vi "4Pi Dual DM - Mode Scan Engine.vi"() -> ()   [LabVIEW 2016]
uses:
  <vilib>/vision/Image Controls.llb/IMAQ Image.ctl
  Hardware Configuration/Hardware Configuration Controls/Device Type.ctl
  Hardware Configuration/Hardware Configuration Controls/Device Function.ctl
  4Pi Dual DM - Controls/4Pi Dual DM - Standard Action.ctl
  4Pi Dual DM - Controls/4Pi Dual DM - Standard Counter Action.ctl
  <vilib>/Analysis/baseanly.llb/Mean (DBL).vi
  <vilib>/Analysis/NI_AALBase.lvlib
  <vilib>/Analysis/NI_AALPro.lvlib
  <vilib>/Analysis/6fits.llb/Curve Fitting Criteria.ctl
  <vilib>/gmath/NI_Gmath.lvlib
panel:
  in  "Image Delay":u32=1
  in  "Accums":u16=1
  in  "Initial Guess":T1={"Amp"=7.0, "Center"=7.0, "Sigma"=7.0, "Offset"=7.0}
  in  "Manual Initial Guess":bool
  in  "Upper Limit":dbl=7.0
  in  "Lower Limit":dbl=7.0
  out "Metric":cluster{dbl[], dbl[]}[](graph)
  out "Image":u16[][](graph)
  in  "Step Size (nm)":u16=7
  in  "Number of Steps":u16=7
  in  "Get Image":bool
  in  "Scan Next Mode":bool
  in  "Metric":u16(ring) items=["Max Intensity", "No Zero Mean", "Threshold Mean"]
  in  "Fit Type":u16(ring) items=["Guassian", "Quadratic"]
  in  "Mode":i32(ring) items=["1", "2", "3", "4", "5", "6", "7", "8", "9", "10", "11", "12", "13", "14", "15", "16", "17", "18", "19", "20", "21", "22", "23", "24", "25", "26", "27", "28", "29", "30", "31", "32", "33", "34", "35", "36", "37", "38", "39", "40", "41", "42", "43", "44", "45", "46", "47", "48", "49", "50", "51", "52", "53", "54", "55", "56", "57", "58", "59", "60", "61", "62", "63", "64", "65", "66", "67", "68", "69", "70", "71", "72", "73", "74", "75", "76", "77", "78", "79", "80", "81", "82", "83", "84", "85", "86", "87", "88", "89", "90", "91", "92", "93", "94", "95", "96", "97", "98", "99", "100", "101", "102", "103", "104", "105", "106", "107", "108", "109", "110", "111", "112", "113", "114", "115", "116", "117", "118", "119", "120", "121", "122", "123", "124", "125", "126", "127", "128", "129", "130", "131", "132", "133", "134", "135", "136", "137", "138", "139", "140", "<141>", "<142>", "<143>", "<144>"]
  in  "Apply":bool
  in  "Fit Data":bool
  in  "Scan Mode":bool
  in  "Exit":bool
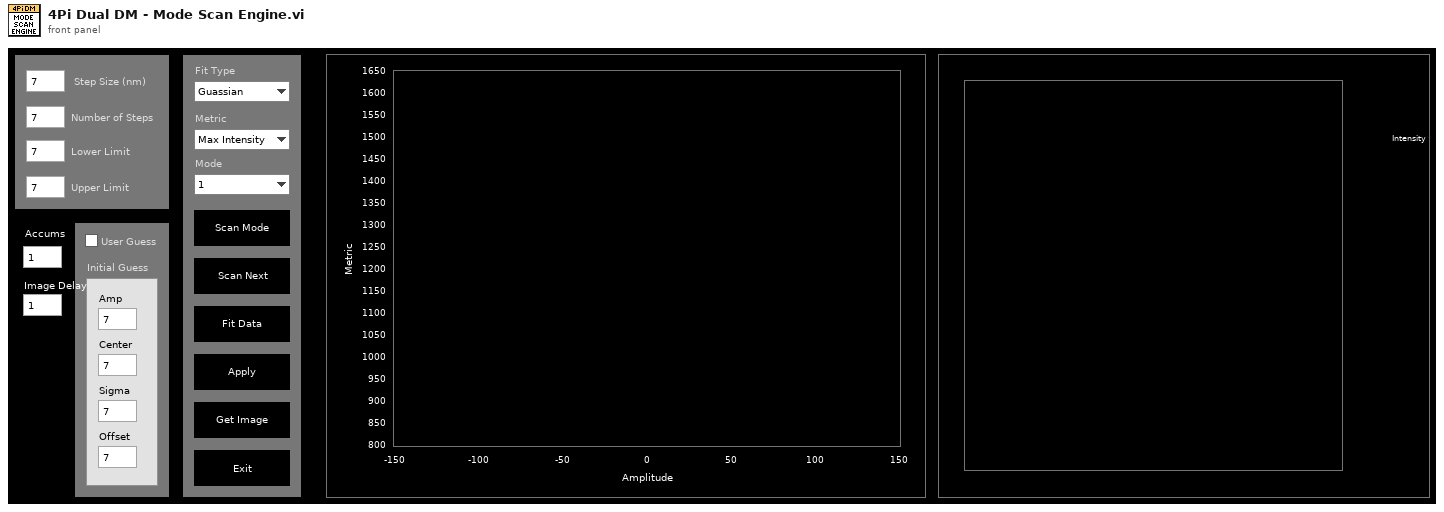
[diagram p1: front panel]
types:
  T1 = cluster{"Amp":dbl, "Center":dbl, "Sigma":dbl, "Offset":dbl}
  T2 = typedef "Device Function.ctl" = enum16{"Primary", "Secondary", "Overview", "Wide Field Drift Correction", "642 nm Excitation", "560 nm Excitation", "546 nm Excitation", "488 nm Excitation", "405 nm Excitation", "Objective Drift Correction", "Objective XY", "Objective Z", "Sample XY", "Sample Coarse Z", "Sample Z", "4Pi Lower", "4Pi Upper", "Adj Cavity"}
  T3 = typedef "Device Type.ctl" = enum16{"AOTF", "Camera", "Deformable Mirror", "Laser", "Shutter", "Stage"}
  T4 = typedef "IMAQ Image.ctl" = refnum<image>
  T5 = typedef "4Pi Dual DM - Standard Action.ctl" = enum16{"Read", "Write"}
  T6 = typedef "4Pi Dual DM - Standard Counter Action.ctl" = enum16{"Initialize", "Update Count", "Get Count"}
  T7 = cluster{"amp min":dbl, "amp max":dbl, "center min":dbl, "center max":dbl, "deviation min":dbl, "deviation max":dbl, "offset min":dbl, "offset max":dbl}
  T8 = enum16{"Linear", "Polynomial", "Exponential", "Power"}
  T9 = typedef "4Pi Dual DM - Mirror Modes DUAL.ctl" = cluster{"Mode":string, "Amplitude":dbl}[][]
  T10 = cluster{"Amplitude Out":dbl[], "Metric Out":dbl[]}
  T11 = cluster{"Amp":dbl, "Numeric":dbl, "Sigma":dbl, "Offset":dbl}
  T12 = typedef "NI_AALPro.lvlib/Curve Fitting Criteria.ctl" = u16
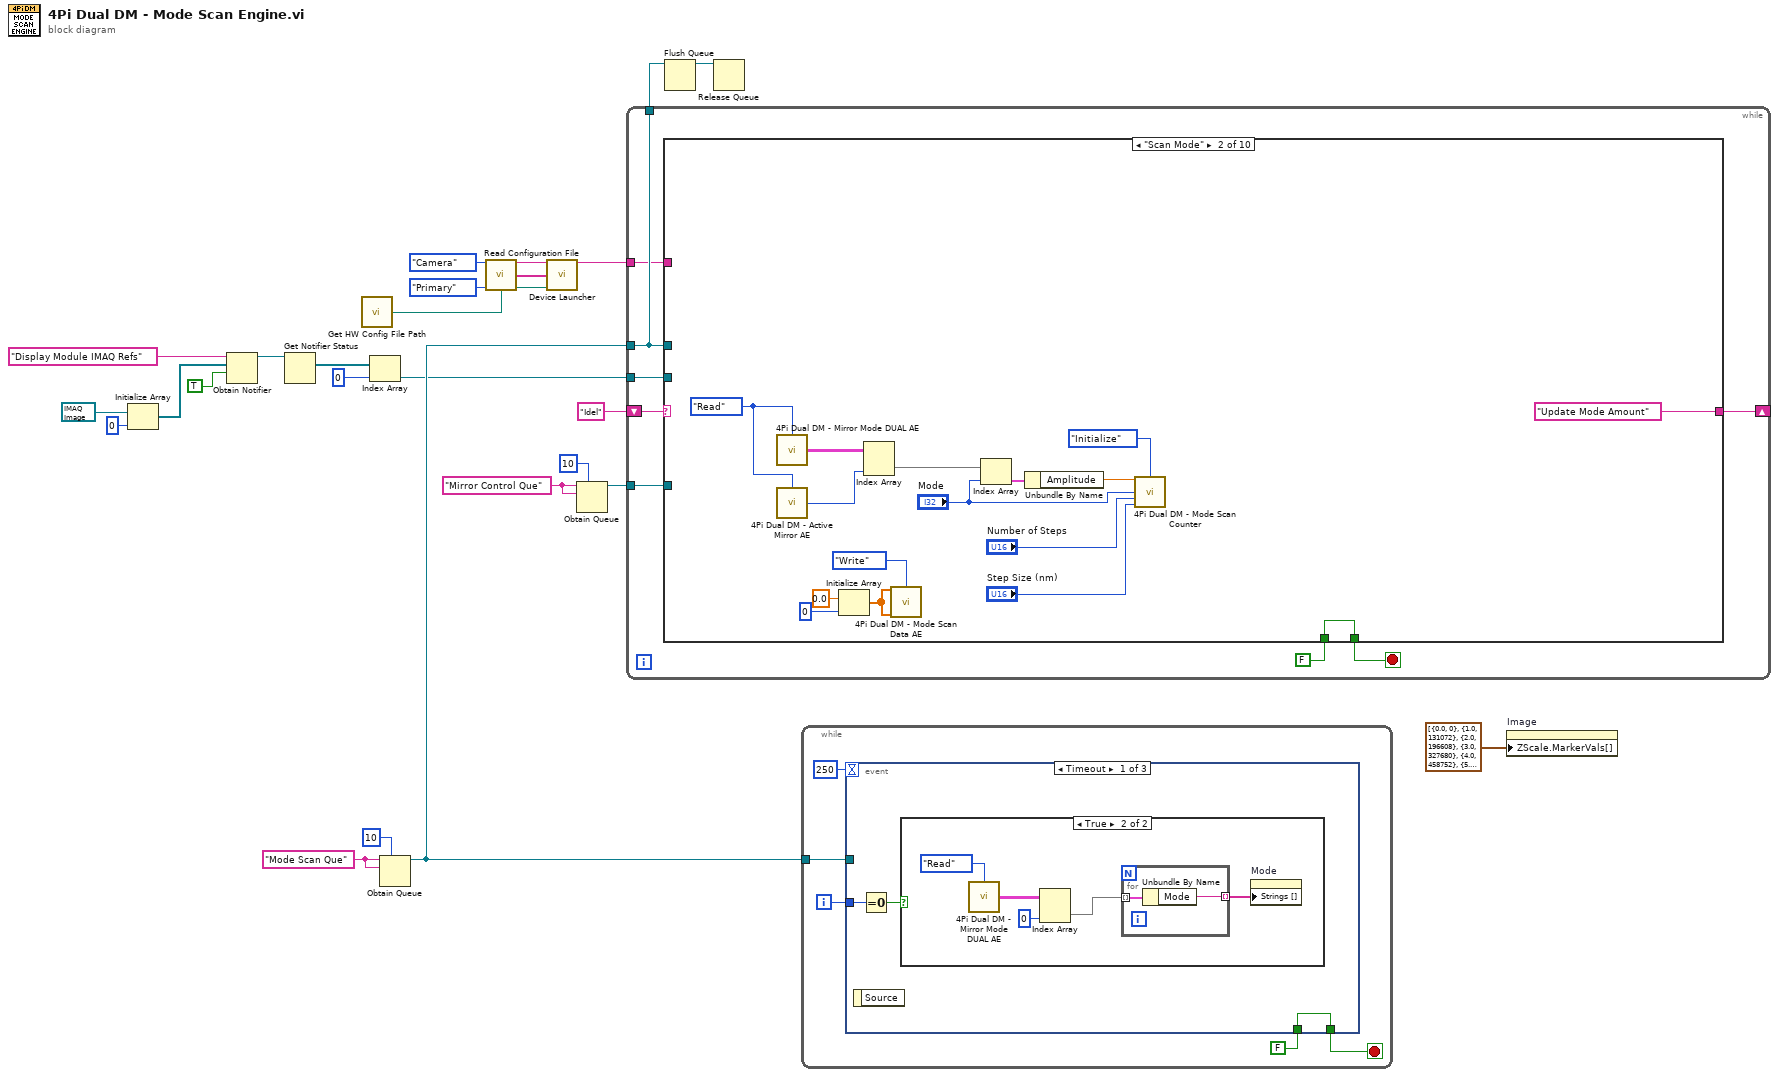
[diagram p0: block diagram]
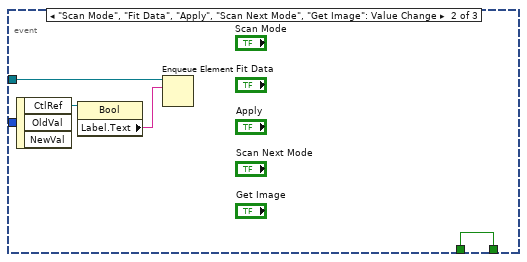
[diagram p3: hidden frame]
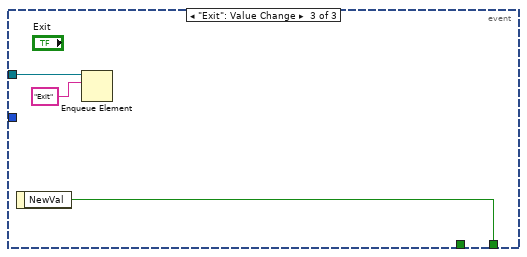
[diagram p4: hidden frame]
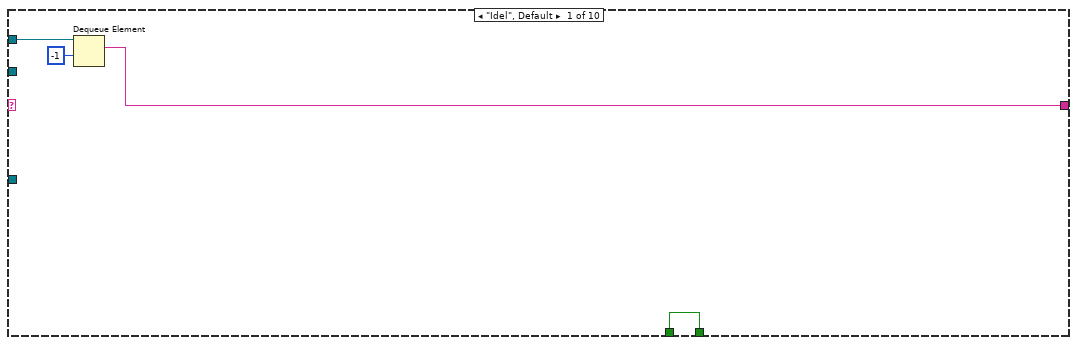
[diagram p5: hidden frame]
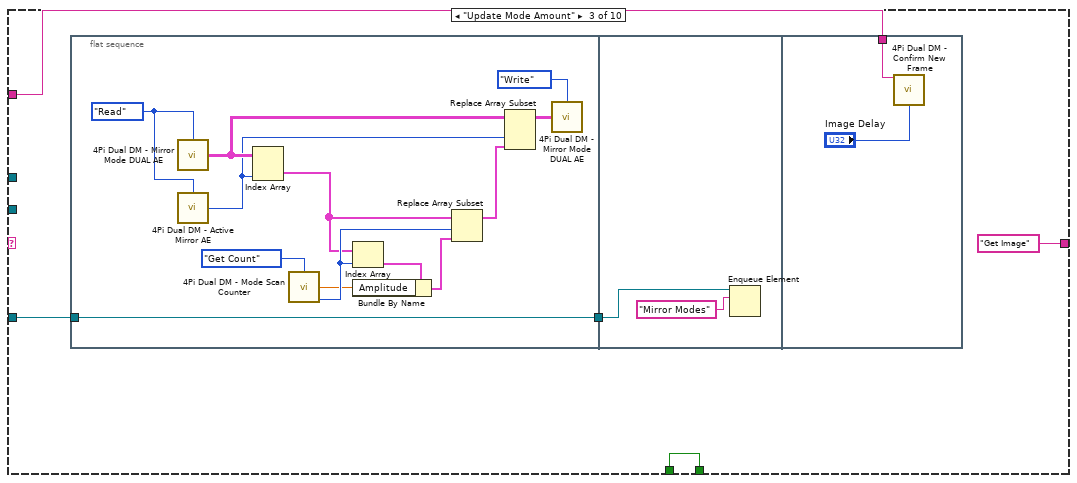
[diagram p6: hidden frame]
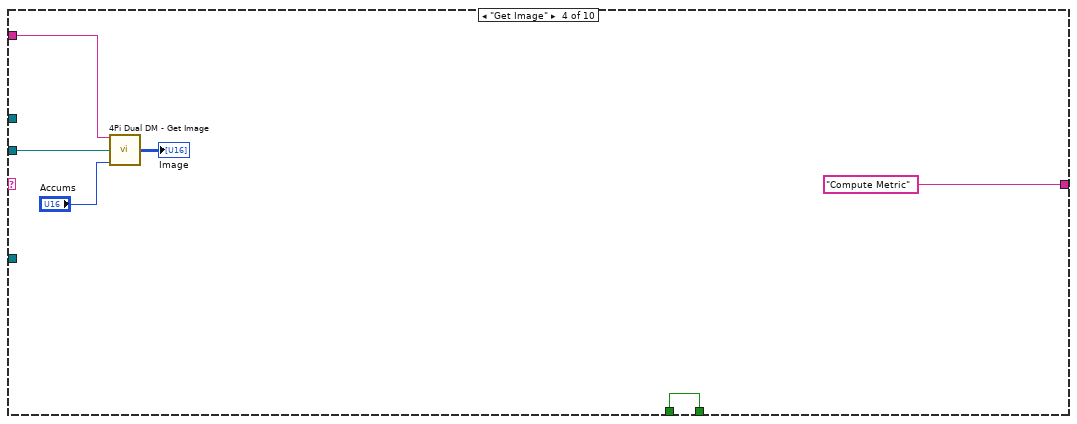
[diagram p7: hidden frame]
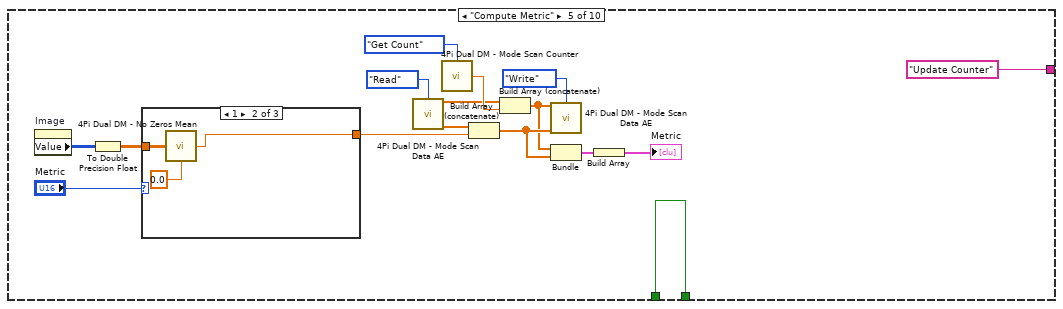
[diagram p8: hidden frame]
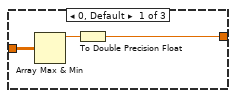
[diagram p9: hidden frame]
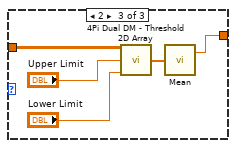
[diagram p10: hidden frame]
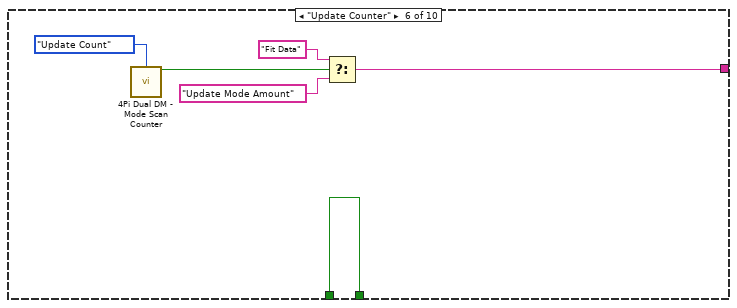
[diagram p11: hidden frame]
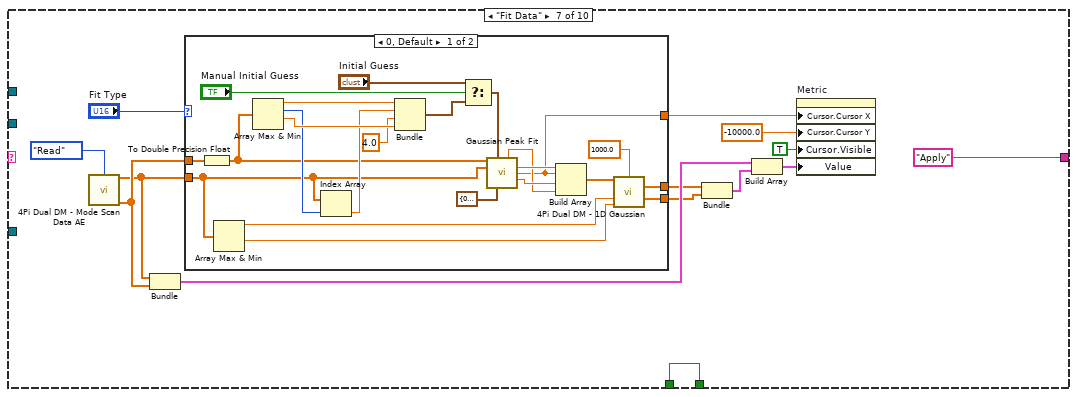
[diagram p12: hidden frame]
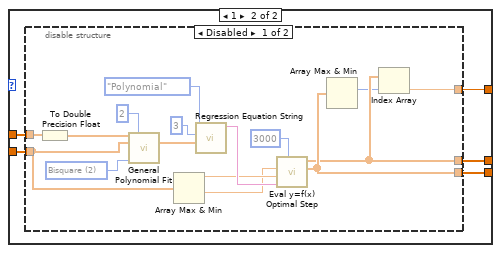
[diagram p13: hidden frame]
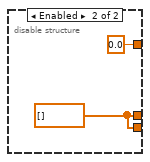
[diagram p14: hidden frame]
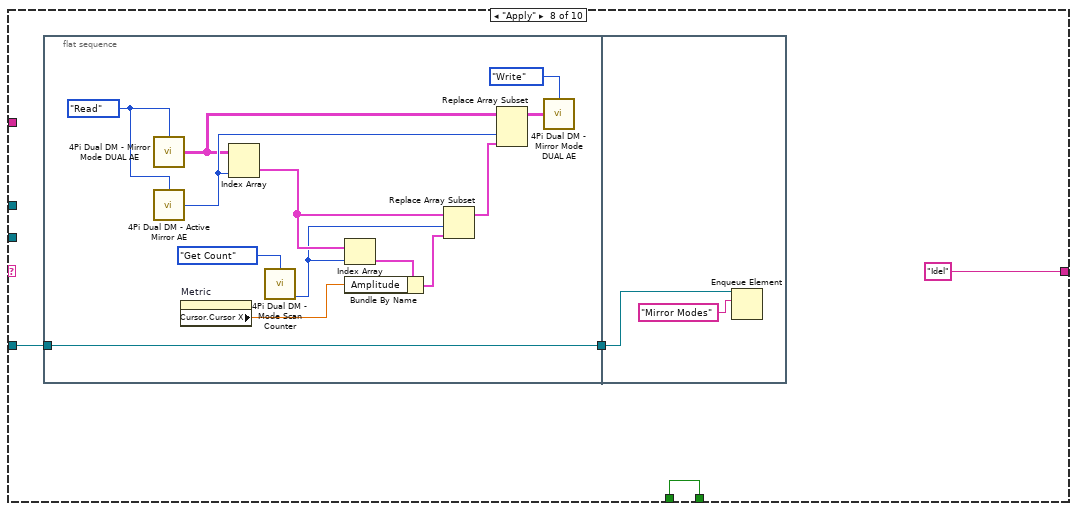
[diagram p15: hidden frame]
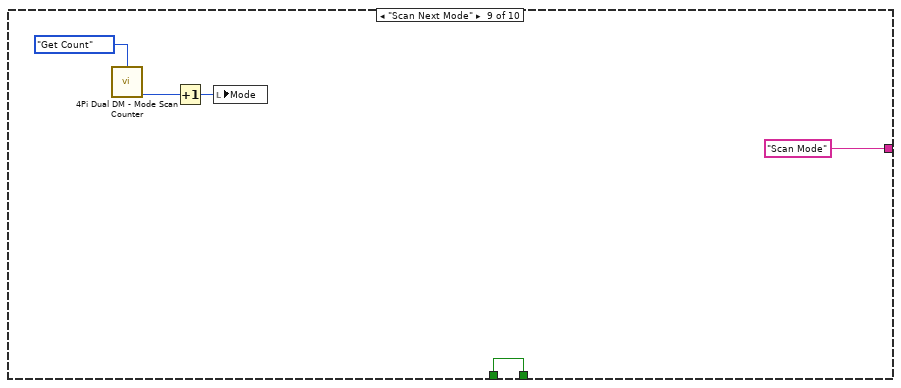
[diagram p16: hidden frame]
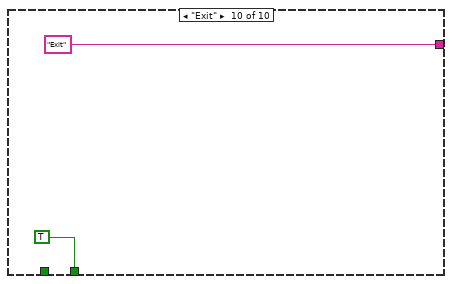
[diagram p17: hidden frame]
diagram:
  w20 = "Mirror Control Que" ("name (unnamed)")
  w25 = "Mode Scan Que" ("name (unnamed)")
  n1 = Initialize Array(T4 refnum ("New Image"), 0 ("dimension size")) -> (w12:T4[])
  n2 = Obtain Notifier(name (unnamed)="Display Module IMAQ Refs", notification data type=w12, create if not found? (T)=TRUE) -> (notifier out=w11:refnum<notifier>)  [unwired: 1 in, 2 out]
  n3 = Get Notifier Status(notifier=w11) -> (current notification=w10:T4[])  [unwired: 1 in, 4 out]
  n4 = call "Get HW Config File Path.vi"() -> ("File Path"=w2:path)  [unwired: 14 in, 1 out]
  n5 = Index Array(array=w10, index=0) -> (element=w8:T4)
  n6 = Obtain Queue(max queue size (-1, unlimited)=10, name (unnamed)=w25, element data type=w25) -> (queue out=w23:refnum<queue>)  [unwired: 2 in, 2 out]
  n7 = call "Read Configuration File.vi"("Device Type"=Device_Type."Camera", "Device Function"=Device_Function."Primary", "Config File Path"=w2) -> ("Unique Notifier Name"=w3:string, "Device Ports/IDs/Channels"=w5:string[], "Device Engine Path"=w4:path)  [unwired: 9 in, 1 out]
  n8 = call "Device Launcher.vi"("Notifier Name"=w3, "Device Ports/IDs/Channels"=w5, "Device Engine Path"=w4) -> ("Notifier Name"=w1:string)  [unwired: 11 in, 1 out]
  n9 = Obtain Queue(max queue size (-1, unlimited)=10, name (unnamed)=w20, element data type=w20) -> (queue out=w18:refnum<queue>)  [unwired: 2 in, 2 out]
  n10 = while {
    shift-right: [w31] -> _
    shift-left: "Idel" -> [w34]
    tunnel: w23 -> [w30]
    tunnel: [w30] -> w22
    tunnel: w18 -> [w29]
    tunnel: w8 -> [w28]
    tunnel: w1 -> [w27]
    stop <- w33 stop-if-true
    n11 = case shown="\"Scan Mode\"" w34 {
      tunnel: [w38 w54 w59 w82 w97 w115 w129 w179 w199 TRUE] -> w33
      tunnel: FALSE -> [w38 w54 w59 w82 w97 w115 w129 w179 w199 _]
      tunnel: w30 -> [w36 _ _ _ _ _ _ _ _ _]
      tunnel: [w35 "Update Mode Amount" ("name (unnamed)") "Get Image" ("name (unnamed)") "Compute Metric" ("name (unnamed)") "Update Counter" ("name (unnamed)") w112 "Apply" ("name (unnamed)") "Idel" ("name (unnamed)") "Scan Mode" ("name (unnamed)") "Exit" ("name (unnamed)")] -> w31
      tunnel: w29 -> [_ _ w58 _ _ _ _ w177 _ _]
      tunnel: w28 -> [_ _ _ w79 _ _ _ _ _ _]
      tunnel: w27 -> [_ _ w55 w78 _ _ _ _ _ _]
      frame "Idel", Default {
        n12 = Dequeue Element(queue=w36, timeout in ms (-1)=-1) -> (element=w35:string)  [unwired: 1 in, 3 out]
      }
      frame "Scan Mode" {
        w41 = 4Pi_Dual_DM_-_Standard_Action."Read" ("Action")
        n13 = call "4Pi Dual DM - Mirror Mode DUAL AE.vi"("Action"=w41) -> ("Mirror Modes Out"=w43:T9)  [unwired: 14 in]
        n14 = call "4Pi Dual DM - Active Mirror AE.vi"("Action"=w41) -> ("Active Mirror"=w42:i32)  [unwired: 14 in]
        n15 = Initialize Array(0.0 ("element"), 0 ("dimension size")) -> (w44:dbl[])
        n16 = Index Array(array=w43, index (col)=w42) -> (element=w40:cluster{"Mode":string, "Amplitude":dbl}[])  [unwired: 1 in]
        n17 = call "4Pi Dual DM - Mode Scan Data AE.vi"("Amplitude"=w44, "Action"=4Pi_Dual_DM_-_Standard_Action."Write", "Metric"=w44) -> ()  [unwired: 11 in, 2 out]
        n18 = Index Array(array=w40, index="Mode") -> (element=w50:cluster{"Mode":string, "Amplitude":dbl})
        n19 = Unbundle By Name(w50) -> ("Amplitude"=w51:dbl)
        n20 = call "4Pi Dual DM - Mode Scan Counter.vi"("Center Value"=w51, "Action"=4Pi_Dual_DM_-_Standard_Counter_Action."Initialize", "Mode"="Mode", "Number of Steps"="Number of Steps", "Step Size"="Step Size (nm)") -> ()  [unwired: 8 in, 3 out]
      }
      frame "Update Mode Amount" {
        n21 = flat-sequence {
          tunnel: w58 -> [w70]
          tunnel: [w70] -> w56
          tunnel: w56 -> [w73]
          tunnel: w55 -> [w75]
          frame #0 {
            w66 = 4Pi_Dual_DM_-_Standard_Action."Read" ("Action")
            n22 = call "4Pi Dual DM - Mirror Mode DUAL AE.vi"("Action"=w66) -> ("Mirror Modes Out"=w63:T9)  [unwired: 14 in]
            n23 = call "4Pi Dual DM - Active Mirror AE.vi"("Action"=w66) -> ("Active Mirror"=w60:i32)  [unwired: 14 in]
            n24 = Index Array(array=w63, index (col)=w60) -> (element=w65:cluster{"Mode":string, "Amplitude":dbl}[])  [unwired: 1 in]
            n25 = call "4Pi Dual DM - Mode Scan Counter.vi"("Action"=4Pi_Dual_DM_-_Standard_Counter_Action."Get Count") -> ("Mode Amount"=w67:dbl, "Current Mode"=w68:i32)  [unwired: 12 in, 1 out]
            n26 = Index Array(array=w65, index=w68) -> (element=w71:cluster{"Mode":string, "Amplitude":dbl})
            n27 = Bundle By Name(cluster=w71, "Amplitude"=w67) -> (w72:cluster{"Mode":string, "Amplitude":dbl})
            n28 = Replace Array Subset(array=w65, new element=w72, index=w68) -> (w61:cluster{"Mode":string, "Amplitude":dbl}[])
            n29 = Replace Array Subset(array=w63, new element=w61, index (col)=w60) -> (w62:T9)  [unwired: 1 in]
            n30 = call "4Pi Dual DM - Mirror Mode DUAL AE.vi"("Action"=4Pi_Dual_DM_-_Standard_Action."Write", "Mirror Modes In"=w62) -> ()  [unwired: 13 in, 1 out]
          }
          frame #1 {
            n31 = Enqueue Element(queue=w73, element="Mirror Modes" ("name (unnamed)")) -> ()  [unwired: 2 in, 3 out]
          }
          frame #2 {
            n32 = call "4Pi Dual DM - Confirm New Frame.vi"("Camera Notifier Name"=w75, "Wait No. (1)"="Image Delay") -> ()  [unwired: 13 in, 1 out]
          }
        }
      }
      frame "Get Image" {
        n33 = call "4Pi Dual DM - Get Image.vi"("Camera Notifier Name"=w78, "Image Ref"=w79, "Frame Accums."="Accums") -> ("Image Out"=→"Image":u16[][])  [unwired: 12 in]
      }
      frame "Compute Metric" {
        n34 = property on="Image" class="IntGraph (strict)"() -> ("Value"=w84:u16[][])  [unwired: 2 in, 2 out]
        n35 = To Double Precision Float(number=w84) -> (double precision float=w83:dbl[][])
        n36 = case shown="1" "Metric" {
          tunnel: w83 -> [w101 w104 w109]
          tunnel: [w99 w103 w107] -> w91
          frame 0, Default {
            n37 = Array Max & Min(array=w101) -> (max value=w100:dbl)  [unwired: 3 out]
            n38 = To Double Precision Float(number=w100) -> (double precision float=w99:dbl)
          }
          frame 1 {
            n39 = call "4Pi Dual DM - No Zeros Mean.vi"("Image IN"=w104, "STDev Factor"=0.0) -> ("No Zero Mean"=w103:dbl)  [unwired: 13 in]
          }
          frame 2 {
            n40 = call "4Pi Dual DM - Threshold 2D Array.vi"("2D Array IN"=w109, "Upper Limit"="Upper Limit", "Lower Limit"="Lower Limit") -> ("Threshold Array Out"=w108:dbl[])  [unwired: 12 in]
            n41 = call-poly <vilib>:"Mean.vi"("X"=w108) -> ("mean"=w107:dbl)  [unwired: 1 out]
          }
        }
        n42 = call "4Pi Dual DM - Mode Scan Data AE.vi"("Action"=4Pi_Dual_DM_-_Standard_Action."Read") -> ("Amplitude Out"=w88:dbl[], "Metric Out"=w89:dbl[])  [unwired: 13 in]
        n43 = call "4Pi Dual DM - Mode Scan Counter.vi"("Action"=4Pi_Dual_DM_-_Standard_Counter_Action."Get Count") -> ("Mode Amount"=w90:dbl)  [unwired: 12 in, 2 out]
        n44 = Build Array (concatenate)(w89, w91) -> (w94:dbl[])
        n45 = Build Array (concatenate)(w88, w90) -> (w93:dbl[])
        n46 = call "4Pi Dual DM - Mode Scan Data AE.vi"("Amplitude"=w93, "Action"=4Pi_Dual_DM_-_Standard_Action."Write", "Metric"=w94) -> ()  [unwired: 11 in, 2 out]
        n47 = Bundle(w93, w94) -> (w95:cluster{dbl[], dbl[]})  [unwired: 1 in]
        n48 = Build Array(w95) -> (→"Metric":cluster{dbl[], dbl[]}[])
      }
      frame "Update Counter" {
        n49 = call "4Pi Dual DM - Mode Scan Counter.vi"("Action"=4Pi_Dual_DM_-_Standard_Counter_Action."Update Count") -> ("Scan Done?"=w110:bool)  [unwired: 12 in, 2 out]
        n50 = Select(t="Fit Data", s=w110, f="Update Mode Amount") -> (s? t:f=w112:string)
      }
      frame "Fit Data" {
        n51 = call "4Pi Dual DM - Mode Scan Data AE.vi"("Action"=4Pi_Dual_DM_-_Standard_Action."Read") -> ("Amplitude Out"=w124:dbl[], "Metric Out"=w125:dbl[])  [unwired: 13 in]
        n52 = Bundle("Amplitude Out"=w124, "Metric Out"=w125) -> (w123:T10)  [unwired: 1 in]
        n53 = case shown="0, Default" "Fit Type" {
          tunnel: w124 -> [w145 w157]
          tunnel: w125 -> [w152 w156]
          tunnel: [w133 w153] -> w118
          tunnel: [w132 w154] -> w121
          tunnel: [w131 w155] -> w120
          frame 0, Default {
            n54 = To Double Precision Float(number=w152) -> (double precision float=w146:dbl[])
            n55 = Array Max & Min(array=w145) -> (max value=w134:dbl, min value=w135:dbl)  [unwired: 2 out]
            n56 = Array Max & Min(array=w146) -> (max value=w151:dbl, max index (indices)=w148:i32, min value=w150:dbl)  [unwired: 1 out]
            n57 = Index Array(array=w145, index=w148) -> (element=w147:dbl)
            n58 = Bundle(w151, "Numeric"=w147, 4.0, w150) -> (w144:cluster{dbl, "Numeric":dbl, dbl, dbl})  [unwired: 1 in]
            n59 = Select(t="Initial Guess", s="Manual Initial Guess", f=w144) -> (s? t:f=w143:T11)
            n60 = call <vilib>:"Gaussian Peak Fit.vi"("Y"=w146, "initial guess"=w143, "X"=w145, "parameter bounds"=T7 {"amp min"=0.0, "amp max"=100000.0, "center min"=-100.0, "center max"=100.0, "deviation min"=0.0, "deviation max"=1000.0, "offset min"=0.0, "offset max"=1000.0}) -> ("offset"=w138:dbl, "amplitude"=w140:dbl, "center"=w133:dbl, "standard deviation"=w139:dbl)  [unwired: 5 in, 3 out]
            n61 = Build Array(w140, w133, w139, w138) -> (w137:dbl[])
            n62 = call "4Pi Dual DM - 1D Gaussian.vi"("Parameters In"=w137, "Number of Points"=1000.0, "Max X Value"=w134, "Min X Value"=w135) -> ("X Values"=w132:dbl[], "Y Values"=w131:dbl[])  [unwired: 10 in]
          }
          frame 1 {
            n63 = disable-structure shown="Disabled" {
              disable-tunnel: w157 -> [w163 _]
              disable-tunnel: w156 -> [w162 _]
              disable-tunnel: [w161 w174] -> w155
              disable-tunnel: [w160 w174] -> w154
              disable-tunnel: [w159 0.0] -> w153
              frame Disabled {
                w172 = T12 2 items=["Least Square", "Least Absolute Residual", "Bisquare"] ("method")
                n64 = To Double Precision Float(number=w162) -> (double precision float=w173:dbl[])
                n65 = call <vilib>:"General Polynomial Fit.vi"("Y"=w173, "polynomial order"=2, "X"=w163, "method"=w172) -> ("Polynomial Coefficients"=w169:dbl[])  [unwired: 8 in, 3 out]
                n66 = Array Max & Min(array=w163) -> (max value=w165:dbl, min value=w164:dbl)  [unwired: 2 out]
                n67 = call "Regression Equation String.vi"("coefficients"=w169, "precision"=3, "fit type"=T8."Polynomial") -> ("Formula"=w167:string)  [unwired: 8 in]
                n68 = call <vilib>:"Eval y=f(x) Optimal Step.vi"("number of points"=u32 3000, "formula"=w167, "end"=w165, "start"=w164) -> ("Y Values"=w161:dbl[], "X Values"=w160:dbl[])  [unwired: 1 in, 2 out]
                n69 = Array Max & Min(array=w161) -> (max index (indices)=w158:i32)  [unwired: 3 out]
                n70 = Index Array(array=w160, index=w158) -> (element=w159:dbl)
              }
              frame Enabled {
                w174 = dbl[] [] ("X Values")
              }
            }
          }
        }
        n71 = Bundle("X Values"=w121, "X Values"=w120) -> (w119:cluster{"X Values":dbl[], "X Values":dbl[]})  [unwired: 1 in]
        n72 = Build Array(w123, w119) -> (w122:cluster{"X Values":dbl[], "X Values":dbl[]}[])
        n73 = property on="Metric" class="XYGraph (strict)"("Cursor.Cursor X"=w118, "Cursor.Cursor Y"=-10000.0 ("Cursor.Cursor Position:Cursor X"), "Cursor.Visible"=TRUE, "Value"=w122) -> ()  [unwired: 2 in, 2 out]
      }
      frame "Apply" {
        n74 = flat-sequence {
          tunnel: w177 -> [w192]
          tunnel: [w192] -> w176
          tunnel: w176 -> [w193]
          frame #0 {
            w184 = 4Pi_Dual_DM_-_Standard_Action."Read" ("Action")
            n75 = call "4Pi Dual DM - Mirror Mode DUAL AE.vi"("Action"=w184) -> ("Mirror Modes Out"=w187:T9)  [unwired: 14 in]
            n76 = call "4Pi Dual DM - Active Mirror AE.vi"("Action"=w184) -> ("Active Mirror"=w190:i32)  [unwired: 14 in]
            n77 = property on="Metric" class="XYGraph (strict)"() -> ("Cursor.Cursor X"=w191:dbl)  [unwired: 2 in, 2 out]
            n78 = Index Array(array=w187, index (col)=w190) -> (element=w185:cluster{"Mode":string, "Amplitude":dbl}[])  [unwired: 1 in]
            n79 = call "4Pi Dual DM - Mode Scan Counter.vi"("Action"=4Pi_Dual_DM_-_Standard_Counter_Action."Get Count") -> ("Current Mode"=w183:i32)  [unwired: 12 in, 2 out]
            n80 = Index Array(array=w185, index=w183) -> (element=w181:cluster{"Mode":string, "Amplitude":dbl})
            n81 = Bundle By Name(cluster=w181, "Amplitude"=w191) -> (w180:cluster{"Mode":string, "Amplitude":dbl})
            n82 = Replace Array Subset(array=w185, new element=w180, index=w183) -> (w189:cluster{"Mode":string, "Amplitude":dbl}[])
            n83 = Replace Array Subset(array=w187, new element=w189, index (col)=w190) -> (w188:T9)  [unwired: 1 in]
            n84 = call "4Pi Dual DM - Mirror Mode DUAL AE.vi"("Action"=4Pi_Dual_DM_-_Standard_Action."Write", "Mirror Modes In"=w188) -> ()  [unwired: 13 in, 1 out]
          }
          frame #1 {
            n85 = Enqueue Element(queue=w193, element="Mirror Modes" ("name (unnamed)")) -> ()  [unwired: 2 in, 3 out]
          }
        }
      }
      frame "Scan Next Mode" {
        n86 = call "4Pi Dual DM - Mode Scan Counter.vi"("Action"=4Pi_Dual_DM_-_Standard_Counter_Action."Get Count") -> ("Current Mode"=w196:i32)  [unwired: 12 in, 2 out]
        n87 = Increment(x=w196) -> (x+1=w197:i32)
        n88 = local write "Mode"(w197) -> ()
      }
      frame "Exit" {
      }
    }
  }
  n89 = Flush Queue(queue=w22) -> (queue out=w21:refnum<queue>)  [unwired: 1 in, 2 out]
  n90 = Release Queue(queue=w21) -> ()  [unwired: 2 in, 3 out]
  n91 = while {
    tunnel: w23 -> [w206]
    i -> [w203]
    stop <- w205 stop-if-true
    n92 = event shown="[0] Timeout" {
      selector: _ -> [_ _ _]
      dyn-events: _ -> [_ _ _]
      timeout: 250 -> [_ _ _]
      tunnel: w206 -> [_ w219 w223]
      tunnel: [w209 w217 w221] -> w205
      tunnel: FALSE -> [w209 w217 _]
      tunnel: w203 -> [w208 _ _]
      event Timeout {
        n93 = event-data() -> ()  [unwired: 1 in, 1 out]
        n94 = Equal To 0?(x=w208) -> (x = 0?=w207:bool)
        n95 = case shown="True" w207 {
          frame False {
          }
          frame True {
            n96 = call "4Pi Dual DM - Mirror Mode DUAL AE.vi"("Action"=4Pi_Dual_DM_-_Standard_Action."Read") -> ("Mirror Modes Out"=w212:T9)  [unwired: 14 in]
            n97 = Index Array(array=w212, index (col)=0 ("disabled index (col)")) -> (element=w210:cluster{"Mode":string, "Amplitude":dbl}[])  [unwired: 1 in]
            n98 = for {
              tunnel: w210 -> [w216] mode=indexing
              tunnel: [w215] -> w214 mode=indexing
              n99 = Unbundle By Name(w216) -> ("Mode"=w215:string)
            }
            n100 = property on="Mode" class="Ring (strict)"("Strings []"=w214) -> ()  [unwired: 2 in, 2 out]
          }
        }
      }
      event "Scan Mode", "Fit Data", "Apply", "Scan Next Mode", "Get Image": Value Change {
        n101 = event-data() -> ("CtlRef"=w218:refnum<vi>)  [unwired: 1 in, 2 out]
        n102 = property class="Bool"(reference=w218) -> ("Label.Text"=w220:string)  [unwired: 1 in, 2 out]
        n103 = Enqueue Element(queue=w219, element=w220) -> ()  [unwired: 2 in, 3 out]
      }
      event "Exit": Value Change {
        n104 = event-data() -> ("NewVal"=w221:bool)  [unwired: 1 in]
        n105 = Enqueue Element(queue=w223, element="Exit") -> ()  [unwired: 2 in, 3 out]
      }
    }
  }
  n106 = property on="Image" class="IntGraph (strict)"("ZScale.MarkerVals[]"=cluster{dbl, u32}[] [{0.0, 0}, {1.0, 131072}, {2.0, 196608}, {3.0, 327680}, {4.0, 458752}, {5.0, 589824}, {6.0, 720896}, {7.0, 851971}, {8.0, 983043}, {9.0, 1114115}, {10.0, 1245187}, {11.0, 1376259}, {12.0, 1507331}, {13.0, 1638403}, {14.0, 1769475}, {15.0, 1769479}, {16.0, 2031623}, {17.0, 2162695}, {18.0, 2293767}, {19.0, 2424839}, {20.0, 2555911}, {21.0, 2686983}, {22.0, 2818055}, {23.0, 2949127}, {24.0, 3080203}, {25.0, 3211275}, {26.0, 3342347}, {27.0, 3473419}, {28.0, 3604491}, {29.0, 3735563}, {30.0, 3866635}, {31.0, 3867403}, {32.0, 4129547}, {33.0, 4260619}, {34.0, 4391691}, {35.0, 4522763}, {36.0, 4653839}, {37.0, 4784911}, {38.0, 4915983}, {39.0, 5178127}, {40.0, 5309199}, {41.0, 5440271}, {42.0, 5571343}, {43.0, 5702415}, {44.0, 5703439}, {45.0, 5965583}, {46.0, 6096655}, {47.0, 6227727}, {48.0, 6358799}, {49.0, 6489871}, {50.0, 6620943}, {51.0, 6752015}, {52.0, 6883087}, {53.0, 7015183}, {54.0, 7146255}, {55.0, 7277327}, {56.0, 7408399}, {57.0, 7539471}, {58.0, 7670543}, {59.0, 7801615}, {60.0, 8063759}, {61.0, 8194831}, {62.0, 8326927}, {63.0, 8457999}, {64.0, 8589075}, {65.0, 8720147}, {66.0, 8851219}, {67.0, 8982291}, {68.0, 9113363}, {69.0, 9114387}, {70.0, 9376531}, {71.0, 9507603}, {72.0, 9638675}, {73.0, 9769747}, {74.0, 9901843}, {75.0, 10032915}, {76.0, 10163987}, {77.0, 10229523}, {78.0, 10295059}, {79.0, 10427155}, {80.0, 10558227}, {81.0, 10689299}, {82.0, 10820371}, {83.0, 10886931}, {84.0, 10952467}, {85.0, 11083539}, {86.0, 11214611}, {87.0, 11215635}, {88.0, 11477779}, {89.0, 11543315}, {90.0, 11608851}, {91.0, 11740947}, {92.0, 11806483}, {93.0, 11872019}, {94.0, 12004115}, {95.0, 12135187}, {96.0, 12266259}, {97.0, 12267283}, {98.0, 12398355}, {99.0, 12529427}, {100.0, 12530451}, {101.0, 12595987}, {102.0, 12530451}, {103.0, 12793619}, {104.0, 12794131}, {105.0, 12794643}, {106.0, 13056787}, {107.0, 13057299}, {108.0, 13057811}, {109.0, 13188883}, {110.0, 13320979}, {111.0, 13386515}, {112.0, 13452563}, {113.0, 13584147}, {114.0, 13584659}, {115.0, 13585171}, {116.0, 13585683}, {117.0, 13717267}, {118.0, 13848339}, {119.0, 13849363}, {120.0, 13849875}, {121.0, 13850387}, {122.0, 13981459}, {123.0, 14113555}, {124.0, 14114067}, {125.0, 14114579}, {126.0, 14115091}, {127.0, 14246675}, {128.0, 14377747}, {129.0, 14378771}, {130.0, 14379283}, {131.0, 14379539}, {132.0, 14379795}, {133.0, 14380819}, {134.0, 14511891}, {135.0, 14643987}, {136.0, 14644503}, {137.0, 14645015}, {138.0, 14645527}, {139.0, 14646039}, {140.0, 14646551}, {141.0, 14778135}, {142.0, 14909207}, {143.0, 14910231}, {144.0, 14910747}, {145.0, 14911259}, {146.0, 14911771}, {147.0, 14912283}, {148.0, 14912797}, {149.0, 15044383}, {150.0, 15175455}, {151.0, 15175967}, {152.0, 15176479}, {153.0, 15176991}, {154.0, 15177507}, {155.0, 15178019}, {156.0, 15178531}, {157.0, 15310115}, {158.0, 15441701}, {159.0, 15441959}, {160.0, 15442215}, {161.0, 15442727}, {162.0, 15443243}, {163.0, 15443755}, {164.0, 15444269}, {165.0, 15444783}, {166.0, 15444783}, {167.0, 15576367}, {168.0, 15707953}, {169.0, 15708467}, {170.0, 15708979}, {171.0, 15708981}, {172.0, 15708983}, {173.0, 15710011}, {174.0, 15710523}, {175.0, 15711037}, {176.0, 15711039}, {177.0, 15711553}, {178.0, 15843139}, {179.0, 15974213}, {180.0, 15974215}, {181.0, 15974217}, {182.0, 15974219}, {183.0, 15975755}, {184.0, 15976271}, {185.0, 15976785}, {186.0, 15977299}, {187.0, 15977301}, {188.0, 15977815}, {189.0, 15978327}, {190.0, 15978331}, {191.0, 16109917}, {192.0, 16241503}, {193.0, 16241505}, {194.0, 16242019}, {195.0, 16242535}, {196.0, 16242537}, {197.0, 16242539}, {198.0, 16243563}, {199.0, 16243567}, {200.0, 16244081}, {201.0, 16244595}, {202.0, 16244599}, {203.0, 16244601}, {204.0, 16244603}, {205.0, 16245627}, {206.0, 16245631}, {207.0, 16245633}, {208.0, 16246147}, {209.0, 16246663}, {210.0, 16377735}, {211.0, 16508811}, {212.0, 16508815}, {213.0, 16509839}, {214.0, 16509843}, {215.0, 16509845}, {216.0, 16509847}, {217.0, 16510361}, {218.0, 16510875}, {219.0, 16510879}, {220.0, 16510881}, {221.0, 16510883}, {222.0, 16511399}, {223.0, 16511911}, {224.0, 16511915}, {225.0, 16511917}, {226.0, 16511919}, {227.0, 16511923}, {228.0, 16512437}, {229.0, 16512951}, {230.0, 16512955}, {231.0, 16512957}, {232.0, 16512959}, {233.0, 16512961}, {234.0, 16512963}, {235.0, 16512967}, {236.0, 16513481}, {237.0, 16513995}, {238.0, 16513999}, {239.0, 16514001}, {240.0, 16514003}, {241.0, 16514005}, {242.0, 16514007}, {243.0, 16514011}, {244.0, 16514013}, {245.0, 16514015}, {246.0, 16514019}, {247.0, 16514021}, {248.0, 16514023}, {249.0, 16514027}, {250.0, 16514029}, {251.0, 16514031}, {252.0, 16514035}, {253.0, 16514037}, {254.0, 16514039}, {255.0, 16514043}] ("Z Scale.Marker Values[]")) -> ()  [unwired: 2 in, 2 out]
